vi "SINGLE DIMENSIONAL ARRAY.vi"() -> ()   [LabVIEW 2019]
panel:
  out "element 2":dbl
  out "element":dbl
  in  "Array":dbl[](array[numeric])
  # "SINGLE DIMENSIONAL ARRAY"
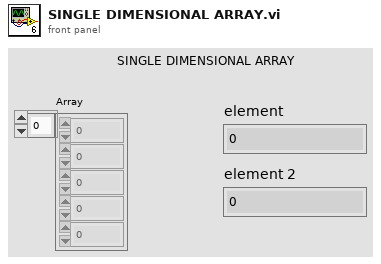
[diagram p1: front panel]
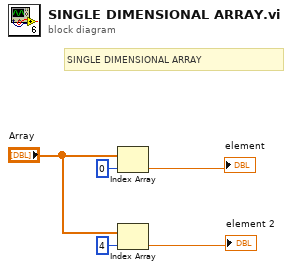
[diagram p0: block diagram]
diagram:
  # "SINGLE DIMENSIONAL ARRAY"
  n1 = Index Array(array="Array", index=0) -> (element=→"element":dbl)
  n2 = Index Array(array="Array", index=4) -> (element=→"element 2":dbl)
